vi "iRobot Navigation Simulator.vi"(8 "stop":bool, 9 "simulation step size (mSec)":u32=5 min=1, 11 "enable 3D visualization?":bool=TRUE) -> (0 "error out":errorcluster, 1 "iRobot Sensors (graphical)":T2 {"Right Wheel (mm/s)" scale=-500.0..500.0; "Left Wheel (mm/s)" scale=-500.0..500.0}, 2 "Diagram Display":picture)   [LabVIEW 2013]
uses:
  iRobot Sensors.ctl
  simulation/Simulate Execution Mode.ctl
panel:
  in  "Tab Control":T1(tab)
  in  "Play":bool
  in  "Wheel Speed (mm/s)":i16(slide)=100 scale=0.0..500.0
  in  "Execution Mode":T4
  in  "C DLL path":path=path "libSimulated iRobot Navigation.dll"
  in  "Tracing On?":bool
  in  "accel smoothing (0-1)":dbl=0.1
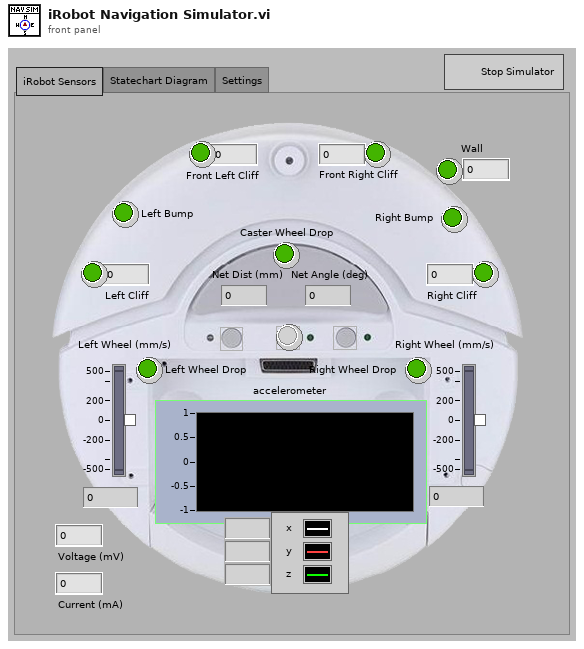
[diagram p1: front panel]
types:
  T1 = enum32{"iRobot Sensors", "Statechart Diagram", "Settings"}
  T2 = typedef "iRobot Sensors.ctl" = cluster{"Caster Wheel Drop":bool, "Left Wheel Drop":bool, "Right Wheel Drop":bool, "Left Bump":bool, "Right Bump":bool, "Left Cliff":bool, "Front Left Cliff":bool, "Front Right Cliff":bool, "Right Cliff":bool, "Wall":bool, "Net Dist (mm)":i32, "Net Angle (deg)":i32, "Wall":u16, "Left Cliff":u16, "Front Left Cliff":u16, "Front Right Cliff":u16, "Right Cliff":u16, "Left Wheel (mm/s)":i16, "Right Wheel (mm/s)":i16, "accelerometer":T3, "Voltage (mV)":dbl, "Current (mA)":dbl}
  T3 = typedef "Accelerometer.ctl" = cluster{"x axis (g)":dbl, "y axis (g)":dbl, "z axis (g)":dbl}
  T4 = typedef "Simulate Execution Mode.ctl" = enum16{"LabVIEW Statechart", "C Statechart"}
  T5 = typedef "Simulate iRobot.ctl" = cluster{"Bump Sensors":refnum<k20>[], "Distance Sensors":refnum<k20>[], "Accelerometer":refnum<k20>, "Wall Sensor":refnum<k20>, "Body":refnum<k20>, "Left Motor":refnum<class "DC Motor Controller.lvclass">, "Right Motor":refnum<class "DC Motor Controller.lvclass">}
  T6 = typedef "iRobot Navigation State Machine.lvsc/Inputs.ctl" = cluster{"net distance (mm)":i32, "net angle (deg)":i32, "Max Wheel Speed (mm/s)":i16, "accelerometer":T3, "iRobot Sensors":T7, "Is Simulator?":bool}
  T7 = typedef "Sensor Group 6.ctl" = cluster{"Bumps + Wheel Drops":T8, "Wall":bool, "Cliff Left":bool, "Cliff Front Left":bool, "Cliff Front Right":bool, "Cliff Right":bool, "Virtual Wall":bool, "Low-Side Driver + Wheel Overcurrent":T9, "Infrared":u8, "Buttons":T10, "Distance (mm)":i32, "Angle (deg)":i32, "Charging State":T11, "Voltage (mV)":u16, "Current (mA)":i16, "Battery Temperature (deg C)":i8, "Battery Charge (mAh)":u16, "Battery Capacity (mAh)":u16, "Wall Signal (0-4095)":u16, "Cliff Left Signal (0-4095)":u16, "Cliff Front Left Signal (0-4095)":u16, "Cliff Front Right Signal (0-4095)":u16, "Cliff Right Signal (0-4095)":u16, "Cargo Bay Digital Inputs":T12, "Cargo Bay Analog Signal (0-1023)":u16, "Charging Sources Available":T13, "OI Mode":T14, "Song Number":u8, "Song Playing":bool, "Number of Stream Packets":u8, "Requested Velocity (mm/s)":i16, "Requested Radius (mm)":i16, "Requested Right Wheel Velocity (mm/s)":i16, "Requested Left Wheel Velocity (mm/s)":i16}
  T8 = typedef "Bumps + Wheel Drops.ctl" = cluster{"Wheeldrop Caster":bool, "Wheeldrop Left":bool, "Wheeldrop Right":bool, "Bump Left":bool, "Bump Right":bool}
  T9 = typedef "Low-Side Driver + Wheel Overcurrent.ctl" = cluster{"Low-Side Driver 0":bool, "Low-Side Driver 1":bool, "Low-Side Driver 2":bool, "Left Wheel":bool, "Right Wheel":bool}
  T10 = typedef "Buttons.ctl" = cluster{"Advance":bool, "Play":bool}
  T11 = typedef "Charging State.ctl" = enum16{"Not Charging", "Reconditioning Charging", "Full Charging", "Trickle Charging", "Waiting", "Charging Fault Condition"}
  T12 = typedef "Cargo Bay Digital Inputs.ctl" = cluster{"Digital Input 0":bool, "Digital Input 1":bool, "Digital Input 2":bool, "Digital Input 3":bool, "Device Detect":bool}
  T13 = typedef "Charging Sources Available.ctl" = cluster{"Internal Charger":bool, "Home Base":bool}
  T14 = typedef "OI Mode.ctl" = enum16{"Off", "Passive", "Safe", "Full"}
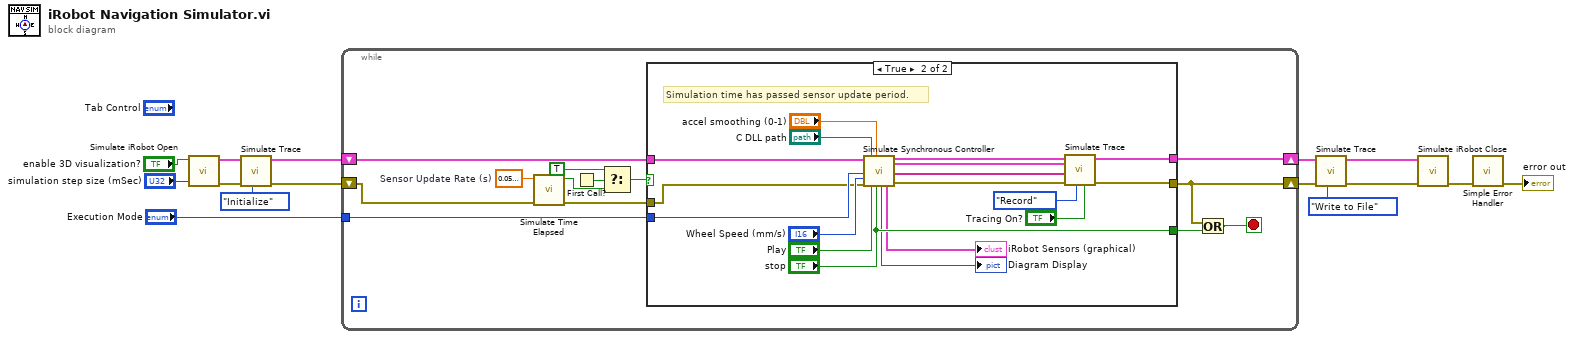
[diagram p0: block diagram]
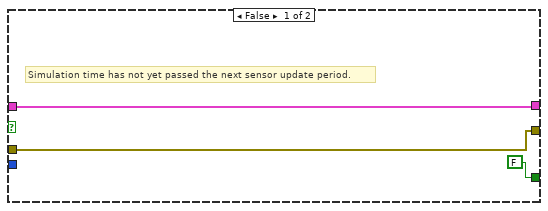
[diagram p2: hidden frame]
diagram:
  n1 = call "Simulate iRobot Open.vi"("step size (mSec)"="simulation step size (mSec)", "enable 3D visualization (T)"="enable 3D visualization?") -> ("error out"=w9:errorcluster, "Cal Climber"=w10:T5)  [unwired: 7 in, 1 out]
  n2 = call "Simulate Trace.vi"("Operation"=enum16{"Initialize", "Record", "Write to File"}."Initialize", "error in (no error)"=w9, "Cal Climber in"=w10) -> ("error out"=w7:errorcluster, "Cal Climber out"=w8:T5)  [unwired: 7 in]
  n3 = while {
    shift-right: [w19] -> w6
    shift-left: w8 -> [w23]
    shift-right: [w17] -> w5
    shift-left: w7 -> [w24]
    tunnel: "Execution Mode" -> [w20]
    stop <- w18 stop-if-true
    w25 = sgl 0.06  # Sensor Update Rate (s)
    n4 = call "Simulate Time Elapsed.vi"("error in (no error)"=w24, "Time Target (s)"=w25) -> ("error out"=w21:errorcluster, "Time Elapsed?"=w26:bool)  [unwired: 7 in, 1 out]
    n5 = First Call?() -> (First Call?: T/F=w28:bool)
    n6 = Select(t=TRUE, s=w28, f=w26) -> (s? t:f=w22:bool)
    n7 = case shown="True" w22 {
      tunnel: w20 -> [_ w49]
      tunnel: [w31 w40] -> w19
      tunnel: [w30 w39] -> w17
      tunnel: w23 -> [w31 w45]
      tunnel: w21 -> [w30 w44]
      tunnel: [FALSE ("stop") "stop"] -> w16
      frame False {
        # "Simulation time has not yet passed the next sensor update period."
      }
      frame True {
        # "Simulation time has passed sensor update period."
        n8 = call "Simulate Synchronous Controller.vi"("Cal Climber in"=w45, "Execution Mode"=w49, "Wheel Speed (mm/s)"="Wheel Speed (mm/s)", "error in (no error)"=w44, "C DLL path"="C DLL path", "Play Button"="Play", "accel smoothing (0-1)"="accel smoothing (0-1)", "Stop Simulation"="stop") -> ("Diagram Display"=→"Diagram Display":picture, "iRobot Sensors (graphical)"=→"iRobot Sensors (graphical)":T2, "Cal Climber out"=w43:T5, "Statechart Inputs"=w42:T6, "Active States"=w33:string[], "error out"=w41:errorcluster)  [unwired: 6 in]
        n9 = call "Simulate Trace.vi"("Tracing On?"="Tracing On?", "Operation"=enum16{"Initialize", "Record", "Write to File"}."Record", "error in (no error)"=w41, "Active States"=w33, "Statechart Inputs"=w42, "Cal Climber in"=w43) -> ("error out"=w39:errorcluster, "Cal Climber out"=w40:T5)  [unwired: 4 in]
      }
    }
    n10 = Or(x=w17, y=w16) -> (x .or. y?=w18:bool)
  }
  n11 = call "Simulate Trace.vi"("Operation"=enum16{"Initialize", "Record", "Write to File"}."Write to File", "error in (no error)"=w5, "Cal Climber in"=w6) -> ("error out"=w3:errorcluster, "Cal Climber out"=w4:T5)  [unwired: 7 in]
  n12 = call "Simulate iRobot Close.vi"("error in"=w3, "Cal Climber"=w4) -> ("error out"=w15:errorcluster)  [unwired: 9 in]
  n13 = call <vilib>:"Simple Error Handler.vi"("error in (no error)"=w15) -> ("error out"=→"error out":errorcluster)  [unwired: 4 in, 4 out]
